vi "UpdateFromActivePrefSet.vi"(8 "error in (no error)":errorcluster, 9 "Active PrefSet":string, 10 "node in":refnum<k20>, 11 "Preferences in":refnum<class "SetListPrefs.lvclass">) -> (0 "error out":errorcluster, 2 "node out":refnum<k20>, 3 "Preferences out":refnum<class "SetListPrefs.lvclass">)   [LabVIEW 2013, in "SetListPrefs.lvclass"]
uses:
  SetListPrefs.lvclass
  SetListPrefs.lvclass/SetListPrefs.ctl
  <vilib>/xml/Close Reference(Node).vi
  <vilib>/xml/NI_XML.lvlib
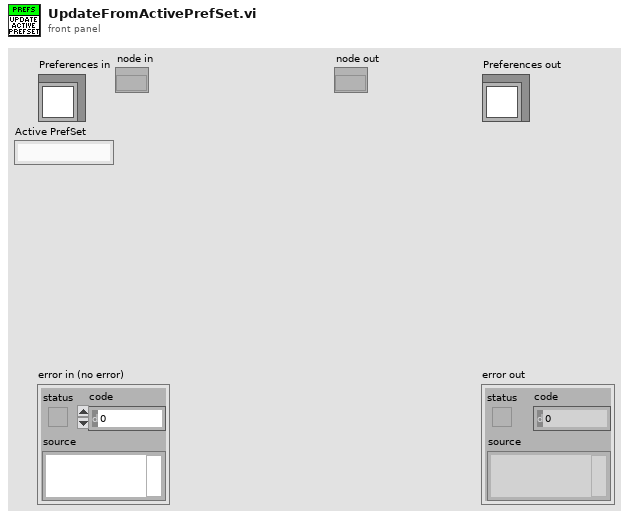
[diagram p1: front panel]
types:
  T1 = typedef "SetListPrefs.lvclass/UpdateResult.ctl" = enum16{"Current", "Old", "Unknown"}
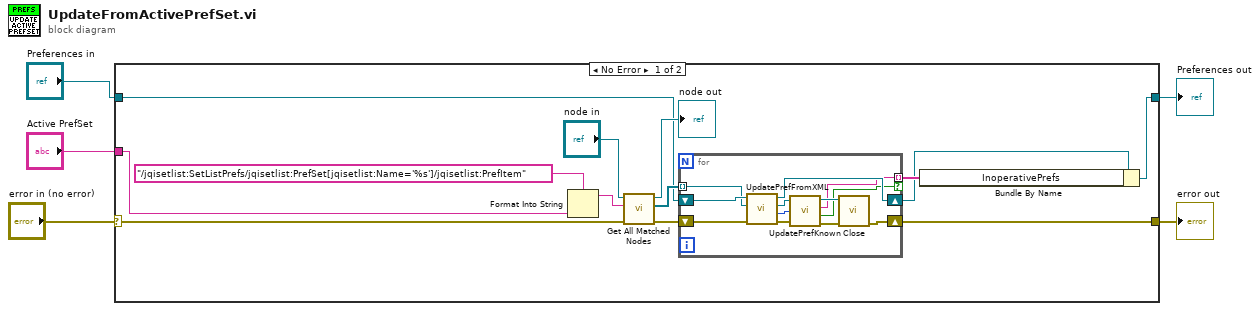
[diagram p0: block diagram]
diagram:
  n1 = case shown="No Error" "error in (no error)" {
    selector: "error in (no error)" -> [w13 w32]
    tunnel: [w6 w32] -> w4
    tunnel: [w10 w31] -> w2
    tunnel: "Preferences in" -> [w7 w31]
    tunnel: "Active PrefSet" -> [w14 _]
    frame No Error {
      n2 = Format Into String(format string="/jqisetlist:SetListPrefs/jqisetlist:PrefSet[jqisetlist:Name='%s']/jqisetlist:PrefItem" ("XPath expression"), w14) -> (resulting string=w15:string)  [unwired: 2 in, 1 out]
      n3 = call <vilib>:"Get All Matched Nodes.vi"("error in (no error)"=w13, "XPath expression"=w15, "node in"="node in") -> ("error out"=w17:errorcluster, "node result array"=w18:refnum<k20>[], "node out"=→"node out":refnum<k20>)  [unwired: 6 in]
      n4 = for {
        tunnel: w18 -> [w21] mode=indexing
        shift-right: [w28] -> w6
        shift-left: w17 -> [w22]
        shift-right: [w29] -> w8
        shift-left: w7 -> [w30]
        tunnel: [w20] -> w9 mode=indexing if=w19
        n5 = call "UpdatePrefFromXML.vi"("error in (no error)"=w22, "PrefItemNode in"=w21, "Preferences in"=w30) -> ("error out"=w25:errorcluster, "UpdateResult"=w26:T1, "PrefItemNode out"=w27:refnum<k20>, "Preferences out"=w29:refnum<class "SetListPrefs.lvclass">)  [unwired: 5 in]
        n6 = call "UpdatePrefKnown.vi"("PrefItemNode in"=w27, "UpdateResult"=w26, "error in (no error)"=w25) -> ("PrefItemNode out"=w23:refnum<k20>, "Updated XML"=w20:string, "Not Current"=w19:bool, "error out"=w24:errorcluster)
        n7 = call-poly <vilib>:"Close.vi"("error in (no error)"=w24, "node"=w23) -> ("error out"=w28:errorcluster)  [unwired: 7 in]
      }
      n8 = Bundle By Name(cluster=w8, "InoperativePrefs"=w9) -> (w10:refnum<class "SetListPrefs.lvclass">)
    }
    frame Error {
    }
  }
  "error out" <- w4
  "Preferences out" <- w2
